vi "5492_ScaleAutoLeft.vi"(10 "Side":string) -> ()   [LabVIEW 2017]
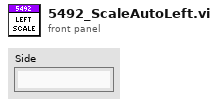
[diagram p1: front panel]
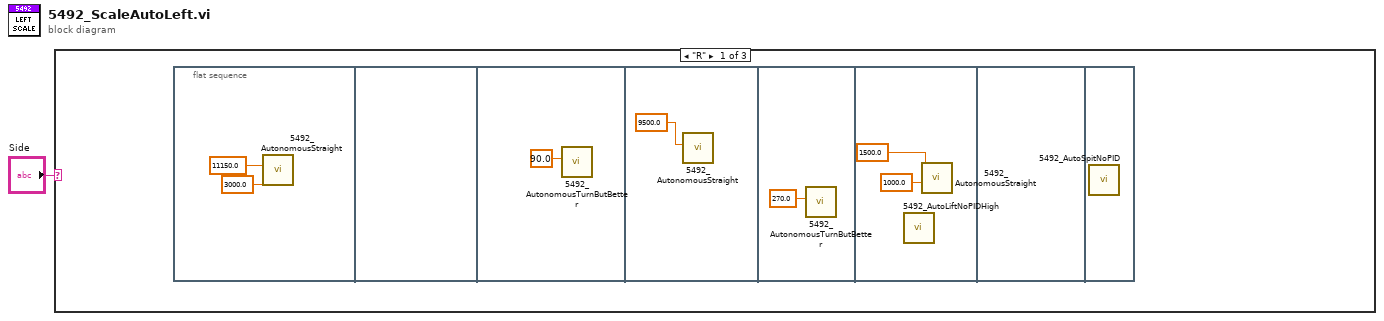
[diagram p0: block diagram]
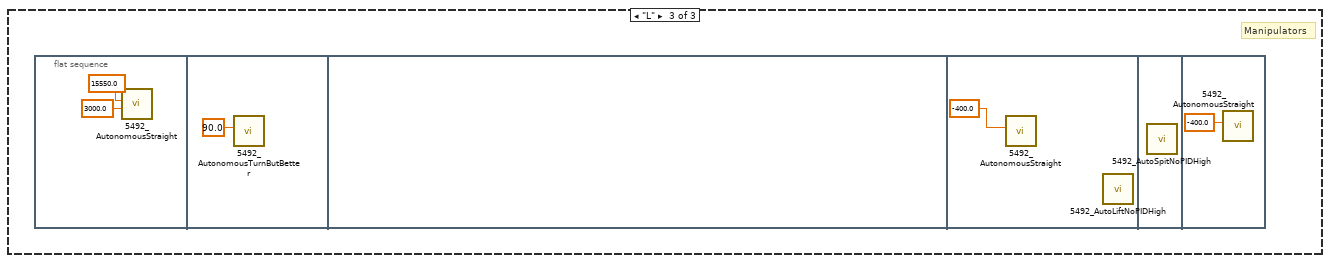
[diagram p3: hidden frame]
diagram:
  n1 = case shown="\"R\"" "Side" {
    frame "R" {
      n2 = flat-sequence {
        frame #0 {
          n3 = call "5492_AutonomousStraight.vi"("Length"=3000.0, "Position Goal"=11150.0) -> ()  [unwired: 9 in, 1 out]
        }
        frame #1 {
        }
        frame #2 {
          n4 = call "5492_AutonomousTurnButBetter.vi"("Yaw Goallll"=90.0) -> ()  [unwired: 10 in, 1 out]
        }
        frame #3 {
          n5 = call "5492_AutonomousStraight.vi"("Position Goal"=9500.0) -> ()  [unwired: 10 in, 1 out]
        }
        frame #4 {
          n6 = call "5492_AutonomousTurnButBetter.vi"("Yaw Goallll"=270.0) -> ()  [unwired: 10 in, 1 out]
        }
        frame #5 {
          n7 = call "5492_AutoLiftNoPIDHigh.vi"() -> ()  [unwired: 12 in]
          n8 = call "5492_AutonomousStraight.vi"("Length"=1000.0, "Position Goal"=1500.0) -> ()  [unwired: 9 in, 1 out]
        }
        frame #6 {
        }
        frame #7 {
          n9 = call "5492_AutoSpitNoPID.vi"() -> ()  [unwired: 12 in]
        }
      }
    }
    frame "What?", Default {
    }
    frame "L" {
      # "Manipulators"
      n10 = flat-sequence {
        frame #0 {
          n11 = call "5492_AutonomousStraight.vi"("Length"=3000.0, "Position Goal"=15550.0) -> ()  [unwired: 9 in, 1 out]
        }
        frame #1 {
          n12 = call "5492_AutonomousTurnButBetter.vi"("Yaw Goallll"=90.0) -> ()  [unwired: 10 in, 1 out]
        }
        frame #2 {
        }
        frame #3 {
          n13 = call "5492_AutonomousStraight.vi"("Position Goal"=-400.0) -> ()  [unwired: 10 in, 1 out]
          n14 = call "5492_AutoLiftNoPIDHigh.vi"() -> ()  [unwired: 12 in]
        }
        frame #4 {
          n15 = call "5492_AutoSpitNoPIDHigh.vi"() -> ()  [unwired: 12 in]
        }
        frame #5 {
          n16 = call "5492_AutonomousStraight.vi"("Position Goal"=-400.0) -> ()  [unwired: 10 in, 1 out]
        }
      }
    }
  }
